vi "Show Points Graph.vi"(0 "Display State In":T1, 5 "Show Points?":bool, 9 "Container State":T2, 11 "error in (no error)":errorcluster) -> (4 "Display State Out":T1, 15 "error out":errorcluster)   [LabVIEW 2009, in "Xgraph simple.xctl"]
doc: "Demonstration of an XControl.\n\nAAL 9/09"
uses:
  Xgraph simple.xctl
  <vilib>/_xctls/Container State.ctl
  Abilities/State Graph.ctl
  <vilib>/_xctls/XControlSupport.lvlib
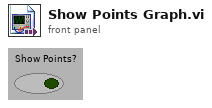
[diagram p1: front panel]
types:
  T1 = typedef "Xgraph simple.xctl/State Graph.ctl" = cluster{"Show Points?":bool}
  T2 = typedef "XControlSupport.lvlib/Container State.ctl" = cluster{"Indicator?":bool, "Run Mode?":bool, " Refnum":refnum<vi>}
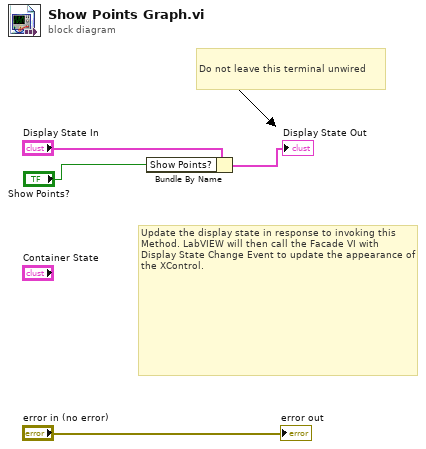
[diagram p0: block diagram]
diagram:
  # "Do not leave this terminal unwired"
  # "Update the display state in response to invoking this Method. LabVIEW will then call the Facade VI with Display State Change Event to update the appearance of the XControl."
  n1 = Bundle By Name(cluster="Display State In", "Show Points?"="Show Points?") -> (→"Display State Out":T1)
  "error out" <- "error in (no error)"
